vi "SetTxOn.vi"(6 "Legacy (f)?":bool, 8 "error in (no error)":errorcluster, 10 "TxOn":bool[](array[boolean])) -> (0 "error out":errorcluster, 5 "Timed Out?":bool)   [LabVIEW 2011]
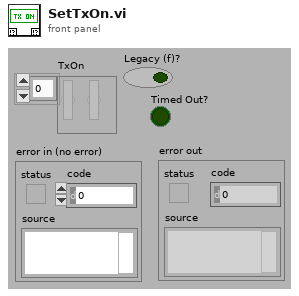
[diagram p1: front panel]
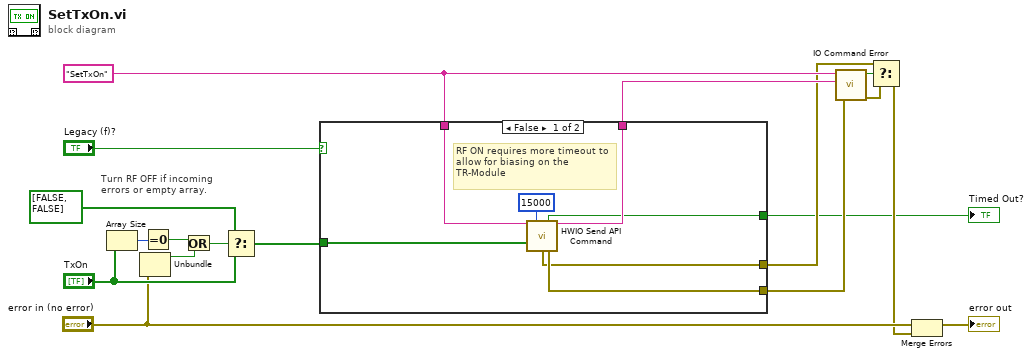
[diagram p0: block diagram]
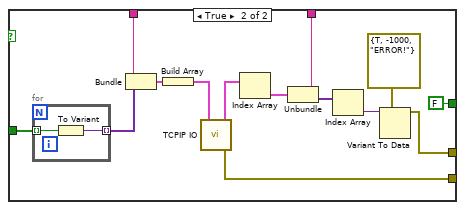
[diagram p2: hidden frame]
diagram:
  w18 = "SetTxOn"
  # "Turn RF OFF if incoming errors or empty array."
  n1 = Array Size(array="TxOn") -> (size(s)=w12:i32)
  n2 = Unbundle("error in (no error)") -> ("status"=w8:bool)  [unwired: 2 out]
  n3 = Equal To 0?(x=w12) -> (x = 0?=w11:bool)
  n4 = Or(x=w11, y=w8) -> (x .or. y?=w10:bool)
  n5 = Select(t=bool[] [FALSE, FALSE], s=w10, f="TxOn") -> (s? t:f=w14:bool[])
  n6 = case shown="False" "Legacy (f)?" {
    tunnel: w18 -> [w24 w37]
    tunnel: [w23 w36] -> w17
    tunnel: [w25 w32] -> w16
    tunnel: w14 -> [w22 w31]
    tunnel: [w21 w27] -> w3
    tunnel: [w19 FALSE ("Timed Out?")] -> w1
    frame False {
      # "RF ON requires more timeout to allow for biasing on the TR-Module"
      n7 = call "HWIO Send API Command.vi"("Action"=w24, "Timeout ms (5000)"=15000 ("PerCommand Timeout (ms)"), "Boolean"=w22) -> ("Timed Out?"=w19:bool, "Action out"=w25:string, "HWError"=w21:errorcluster, "error out"=w23:errorcluster)  [unwired: 5 in, 4 out]
    }
    frame True {
      n8 = for {
        tunnel: w31 -> [w41] mode=indexing
        tunnel: [w40] -> w39 mode=indexing
        n9 = To Variant(anything=w41) -> (Variant=w40:variant)
      }
      n10 = Bundle(w37, w39) -> (w38:cluster{string, variant[]})  [unwired: 1 out]
      n11 = Build Array(w38) -> (w35:cluster{string, variant[]}[])
      n12 = call "TCPIP IO.vi"("Commands"=w35) -> ("error out"=w36:errorcluster, "Responses"=w33:cluster{string, variant[]}[])  [unwired: 2 in, 3 out]
      n13 = Index Array(array=w33) -> (element=w34:cluster{string, variant[]})  [unwired: 1 in]
      n14 = Unbundle(w34) -> (w32:string, w28:variant[])
      n15 = Index Array(array=w28) -> (element=w30:variant)  [unwired: 1 in]
      n16 = Variant To Data(type=errorcluster {"status"=TRUE, "code"=-1000, "source"="ERROR!"} ("error out"), Variant=w30) -> (data=w27:errorcluster)  [unwired: 1 in, 1 out]
    }
  }
  "Timed Out?" <- w1
  n17 = call "IO Command Error.vi"("error in (no error)"=w17, "Command Returned (\"\")"=w16, "Command Sent (\"\")"=w18) -> ("error out"=w5:errorcluster, "HW ERR?"=w6:bool)  [unwired: 3 out]
  n18 = Select(t=w3, s=w6, f=w5) -> (s? t:f=w4:errorcluster)
  n19 = Merge Errors("error in (no error)", w4) -> (→"error out":errorcluster)
